vi "PicoScopeAdcToVolts.vi"(0 "Max_adc":i16=32767, 2 "Range Index":u16, 3 "Data":i16[](array[numeric])) -> (1 "Data (Volts)":dbl[](array[numeric]))   [LabVIEW 2020]
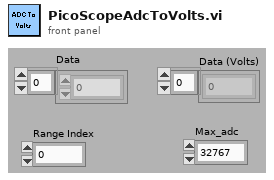
[diagram p1: front panel]
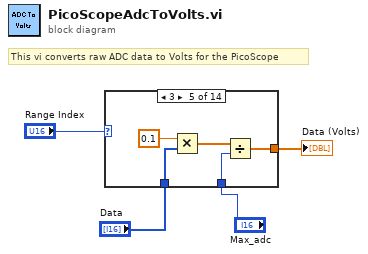
[diagram p0: block diagram]
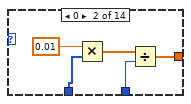
[diagram p3: hidden frame]
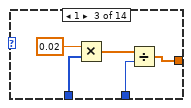
[diagram p4: hidden frame]
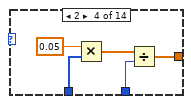
[diagram p5: hidden frame]
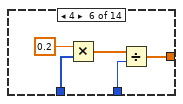
[diagram p6: hidden frame]
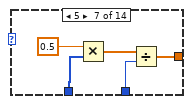
[diagram p7: hidden frame]
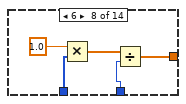
[diagram p8: hidden frame]
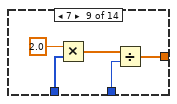
[diagram p9: hidden frame]
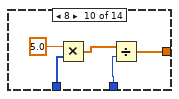
[diagram p10: hidden frame]
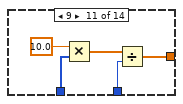
[diagram p11: hidden frame]
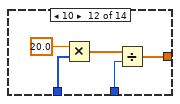
[diagram p12: hidden frame]
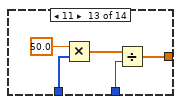
[diagram p13: hidden frame]
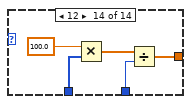
[diagram p14: hidden frame]
diagram:
  # "This vi converts raw ADC data to Volts for the PicoScope"
  n1 = case shown="3" "Range Index" {
    tunnel: [w5 w8 w12 w18 w23 w28 w33 w37 w43 w48 w53 w58 w63 w68] -> w2
    tunnel: "Data" -> [w5 w6 w13 w17 w22 w27 w32 w38 w42 w47 w52 w57 w62 w67]
    tunnel: "Max_adc" -> [_ w7 w11 w16 w21 w26 w31 w36 w41 w46 w51 w56 w61 w66]
    frame Default {
    }
    frame 0 {
      n2 = Multiply(x=0.01, y=w6) -> (x*y=w9:dbl[])
      n3 = Divide(x=w9, y=w7) -> (x/y=w8:dbl[])
    }
    frame 1 {
      n4 = Multiply(x=0.02, y=w13) -> (x*y=w15:dbl[])
      n5 = Divide(x=w15, y=w11) -> (x/y=w12:dbl[])
    }
    frame 2 {
      n6 = Multiply(x=0.05, y=w17) -> (x*y=w19:dbl[])
      n7 = Divide(x=w19, y=w16) -> (x/y=w18:dbl[])
    }
    frame 3 {
      n8 = Multiply(x=0.1, y=w22) -> (x*y=w24:dbl[])
      n9 = Divide(x=w24, y=w21) -> (x/y=w23:dbl[])
    }
    frame 4 {
      n10 = Multiply(x=0.2, y=w27) -> (x*y=w30:dbl[])
      n11 = Divide(x=w30, y=w26) -> (x/y=w28:dbl[])
    }
    frame 5 {
      n12 = Multiply(x=0.5, y=w32) -> (x*y=w35:dbl[])
      n13 = Divide(x=w35, y=w31) -> (x/y=w33:dbl[])
    }
    frame 6 {
      n14 = Multiply(x=1.0, y=w38) -> (x*y=w40:dbl[])
      n15 = Divide(x=w40, y=w36) -> (x/y=w37:dbl[])
    }
    frame 7 {
      n16 = Multiply(x=2.0, y=w42) -> (x*y=w45:dbl[])
      n17 = Divide(x=w45, y=w41) -> (x/y=w43:dbl[])
    }
    frame 8 {
      n18 = Multiply(x=5.0, y=w47) -> (x*y=w50:dbl[])
      n19 = Divide(x=w50, y=w46) -> (x/y=w48:dbl[])
    }
    frame 9 {
      n20 = Multiply(x=10.0, y=w52) -> (x*y=w55:dbl[])
      n21 = Divide(x=w55, y=w51) -> (x/y=w53:dbl[])
    }
    frame 10 {
      n22 = Multiply(x=20.0, y=w57) -> (x*y=w60:dbl[])
      n23 = Divide(x=w60, y=w56) -> (x/y=w58:dbl[])
    }
    frame 11 {
      n24 = Multiply(x=50.0, y=w62) -> (x*y=w65:dbl[])
      n25 = Divide(x=w65, y=w61) -> (x/y=w63:dbl[])
    }
    frame 12 {
      n26 = Multiply(x=100.0, y=w67) -> (x*y=w70:dbl[])
      n27 = Divide(x=w70, y=w66) -> (x/y=w68:dbl[])
    }
  }
  "Data (Volts)" <- w2
